vi "Radians per Second to RPM.vi"   [LabVIEW 2020, in "NI_AngleConversion.lvlib"]
doc: "Converts data from radians per second to revolutions per minute (RPM)."
uses:
  <vilib>/Analysis/NI_AngleConversion.lvlib
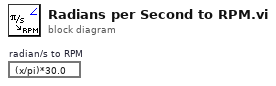
[diagram p0: block diagram]
diagram:
  n1 = expression code="(x/pi)*30.0" "radian/s to RPM"() -> ()  [unwired: 1 in, 1 out]
